vi "Stop The System.vi"(8 "Root Actor Address":refnum<class "Mail Strategy.lvclass">, 11 "System Actor in":refnum<class "System Actor.lvclass">) -> (3 "System Actor Out":refnum<class "System Actor.lvclass">)   [LabVIEW 2024, in "System Actor.lvclass"]
uses:
  System Actor.lvclass
  Messenger/Mail Strategy/Mail Strategy.lvclass
  Message/Message.lvclass
  Message/Type Def/CMD Type.ctl
  Message/Type Def/General CMD.ctl
  Message/Message.lvclass/Message.ctl
  System Actor.lvclass/System Actor.ctl
  Message/Public Data/Write CMD Type.vi
  Message/Public Data/Write General CMD.vi
  Public Data/Call Messenger.vi
  Messenger/Messenger/Messenger.lvclass
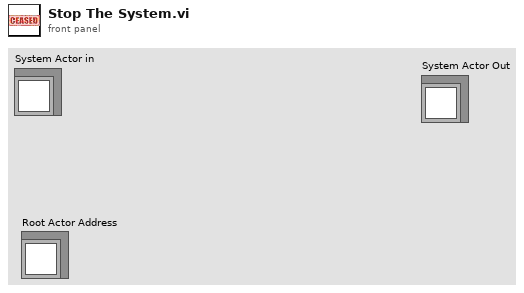
[diagram p1: front panel]
types:
  T1 = typedef "General CMD.ctl" = enum16{"None", "Stop", "Abort", "Running Task", "Running Batch Tasks", "Task Self Running", "Emergency Stop", "Subscribe", "UnSubscribe", "Pause", "Receive Parameters", "Active", "Resume", "De-Activate"}
  T2 = typedef "CMD Type.ctl" = enum16{"None", "General CMD", "1st CMD", "2nd CMD", "3rd CMD", "4th CMD", "5th CMD", "6th CMD", "7th CMD"}
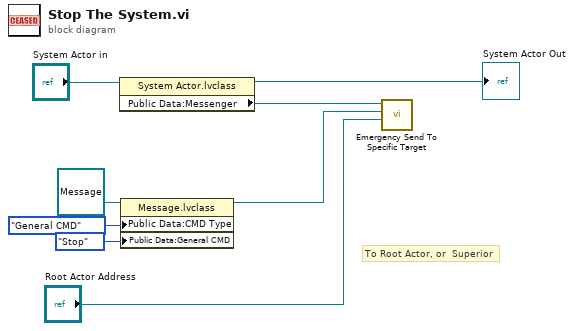
[diagram p0: block diagram]
diagram:
  # "To Root Actor, or  Superior"
  n1 = property class="System Actor.lvclass"(reference="System Actor in") -> (reference out=→"System Actor Out":refnum<class "System Actor.lvclass">, "Public Data:Messenger"=w3:refnum<class "Messenger.lvclass">)  [unwired: 1 in, 1 out]
  n2 = property class="Message.lvclass"(reference=refnum<class "Message.lvclass"> refnum ("Message.lvclass"), "Public Data:CMD Type"=CMD_Type."General CMD" ("CMD Type"), "Public Data:General CMD"=General_CMD."Stop" ("General CMD")) -> (reference out=w5:refnum<class "Message.lvclass">)  [unwired: 1 in, 1 out]
  n3 = call-dynamic "Emergency Send To Specific Target.vi"("Mail Strategy In"="Root Actor Address", "Message In"=w5, "Messenger in"=w3) -> ()  [unwired: 7 in, 2 out]
